vi "setgetScanParameters.vi"(8 "error in":T2, 10 "Set/Get":bool, 11 "Scan Parameters Cluster":T1={"Lines"=-2147483648, "Columns"=-2147483648, "X Range "=-inf, "Y Range "=-inf, "Pixel Size"=-inf, "Origin X"=-inf, "Origin Y"=-inf, "Rotation"=-inf, "Sample Time"=-inf} {"Sample Time" format="%#_g µs"; "Rotation" format="%#_g deg"; "Origin Y" format="%#_g nm"; "Origin X" format="%#_g nm"; "Pixel Size" format="%#_g nm"; "Y Range" format="%#_g nm"; "X Range" format="%#_g nm"; "Columns" max=250; "Lines" max=250}) -> (0 "error out":T2, 2 "IN = OUT?":bool, 3 "Output Cluster":T1={"Lines"=-2147483648, "Columns"=-2147483648, "X Range "=-inf, "Y Range "=-inf, "Pixel Size"=-inf, "Origin X"=-inf, "Origin Y"=-inf, "Rotation"=-inf, "Sample Time"=-inf} {"Sample Time" format="%#_g µs"; "Rotation" format="%#_g deg"; "Origin Y" format="%#_g nm"; "Origin X" format="%#_g nm"; "Pixel Size" format="%#_g nm"; "Y Range" format="%#_g nm"; "X Range" format="%#_g nm"; "Columns" max=250; "Lines" max=250})   [LabVIEW 2016]
doc: "You can set or/and retrieve the values of the scanParameters Cluster. If the input Set/Get equals \"true\" the values of the input cluster will be set. If it equals \"false\" the current values will be retrieved and written into the Output Cluster. The output \"IN = OUT?\" indicates whether the Scan Parameters Cluster equals the Output Cluster. If it is true, you can be sure, that the values you entered into the input-cluster, has been accepted and written to the server."
uses:
  Controls/Scan_Parameters.ctl
  Controls/Error_Out.ctl
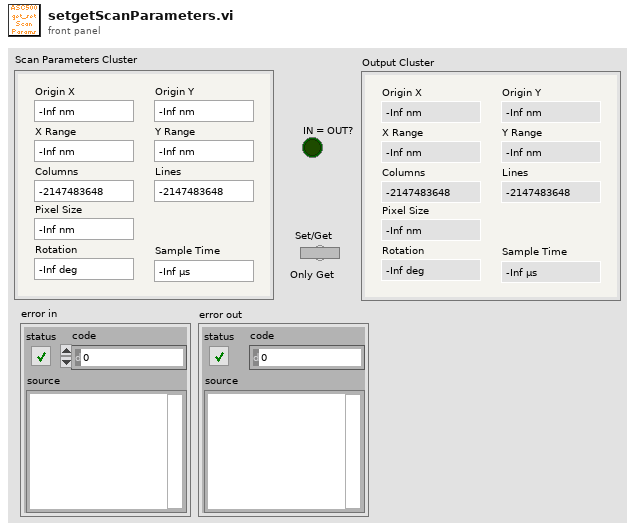
[diagram p1: front panel]
types:
  T1 = typedef "Scan_Parameters.ctl" = cluster{"Lines":i32, "Columns":i32, "X Range ":sgl, "Y Range ":sgl, "Pixel Size":sgl, "Origin X":sgl, "Origin Y":sgl, "Rotation":sgl, "Sample Time":sgl}
  T2 = typedef "Error_Out.ctl" = errorcluster
  T3 = cluster{"Lines":bool, "Columns":bool, "X Range ":bool, "Y Range ":bool, "Pixel Size":bool, "Origin X":bool, "Origin Y":bool, "Rotation":bool, "Sample Time":bool}
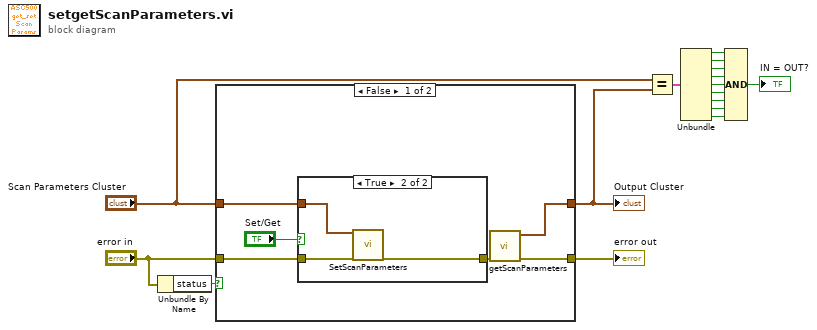
[diagram p0: block diagram]
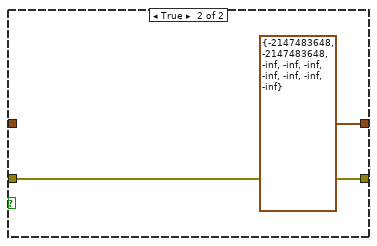
[diagram p3: hidden frame]
diagram:
  n1 = Unbundle By Name("error in") -> ("status"=w14:bool)
  n2 = case shown="False" w14 {
    tunnel: "Scan Parameters Cluster" -> [w22 _]
    tunnel: "error in" -> [w20 w28]
    tunnel: [w17 w28] -> w16
    tunnel: [w18 T1 {"Lines"=-2147483648, "Columns"=-2147483648, "X Range "=-inf, "Y Range "=-inf, "Pixel Size"=-inf, "Origin X"=-inf, "Origin Y"=-inf, "Rotation"=-inf, "Sample Time"=-inf} ("Output Cluster")] -> w13
    frame False {
      n3 = case shown="True" "Set/Get" {
        tunnel: w22 -> [_ w24]
        tunnel: [w23 w26] -> w21
        tunnel: w20 -> [w23 w25]
        frame False {
        }
        frame True {
          n4 = call "SetScanParameters.vi"("Scan Parameters Cluster"=w24, "error in"=w25) -> ("error out"=w26:T2)  [unwired: 16 in, 1 out]
        }
      }
      n5 = call "getScanParameters.vi"("error in"=w21) -> ("error out"=w17:T2, "Output Scan Cluster"=w18:T1)  [unwired: 9 in]
    }
    frame True {
    }
  }
  "Output Cluster" <- w13
  "error out" <- w16
  n6 = Equal?(x="Scan Parameters Cluster", y=w13) -> (x = y?=w2:T3)
  n7 = Unbundle(w2) -> ("Lines"=w11:bool, "Columns"=w10:bool, "X Range"=w9:bool, "Y Range"=w8:bool, "Pixel Size"=w7:bool, "Origin X"=w6:bool, "Origin Y"=w5:bool, "Rotation"=w4:bool, "Sample Time"=w3:bool)
  n8 = Compound Arithmetic op=AND(w11, w10, w9, w8, w7, w6, w5, w4, w3) -> (→"IN = OUT?":bool)
